vi "Read 1D array Shared Variables.vi"(8 "Error In":errorcluster, 9 "Array of Type code":i32[](array[numeric]), 10 "Array of SV Refnums":refnum<k21>[](array[refnum]), 11 "Waveform Array in":waveform(dbl)[][](array[waveform])) -> (0 "Error Out":errorcluster, 3 "Waveform Array out":waveform(dbl)[][](array[waveform]))   [LabVIEW 2014]
doc: "<B>Copyright</B>: (c) MHWirth 2015. All rights are reserved.\n\nThis subVI reads all shared variables (that are of <B>1D array</B>), and consequently updates the input array of waveforms.\n\n<B>Shaved Variable Types</B>:\n1D array of type code 1 to 12 -"
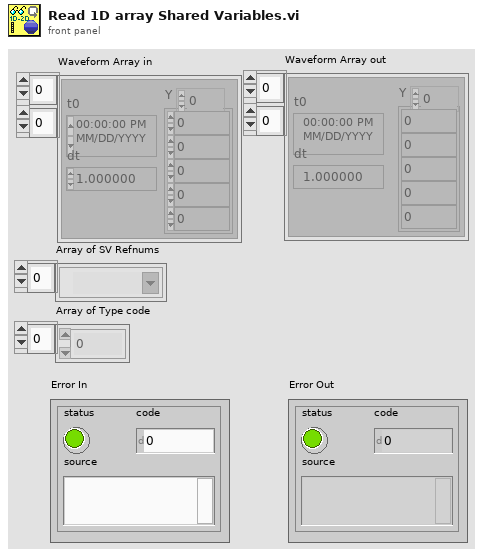
[diagram p1: front panel]
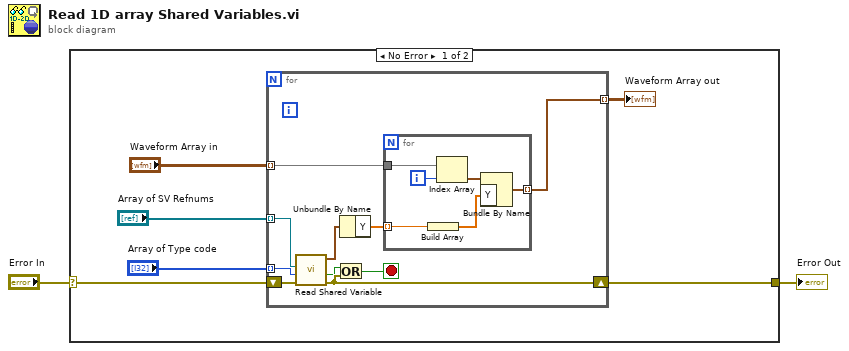
[diagram p0: block diagram]
diagram:
  n1 = case shown="No Error" "Error In" {
    selector: "Error In" -> [w6 w25]
    tunnel: [w5 w25] -> w1
    frame No Error {
      n2 = for {
        tunnel: "Array of SV Refnums" -> [w15] mode=indexing
        tunnel: "Array of Type code" -> [w16] mode=indexing
        shift-right: [w14] -> w5
        shift-left: w6 -> [w17]
        tunnel: "Waveform Array in" -> [w11] mode=indexing
        tunnel: [w9] -> w3 mode=indexing
        stop <- w18 stop-if-true
        n3 = call "Read Shared Variable.vi"("Error In"=w17, "Type code"=w16, "Refnum"=w15) -> ("Error Out"=w14:errorcluster, "status"=w13:bool, "Waveform out"=w12:waveform(dbl))  [unwired: 5 in, 1 out]
        n4 = Or(x=w13, y=w14) -> (x .or. y?=w18:bool)
        n5 = Unbundle By Name(w12) -> ("Y"=w10:dbl[])
        n6 = for {
          tunnel: w11 -> [w20]
          tunnel: w10 -> [w24] mode=indexing
          tunnel: [w22] -> w9 mode=indexing
          i -> [w21]
          n7 = Build Array(w24) -> (w23:dbl[])
          n8 = Index Array(array=w20, index=w21) -> (element=w19:waveform(dbl))
          n9 = Bundle By Name(cluster=w19, "Y"=w23) -> (w22:waveform(dbl))
        }
      }
      "Waveform Array out" <- w3
    }
    frame Error {
    }
  }
  "Error Out" <- w1
